vi "obtain_scanner_values.vi"(8 "error in (no error)":errorcluster, 11 "ScanHeadDL090202 in":refnum<class "ScanHeadDL090202.lvclass">) -> (0 "error out":errorcluster, 1 "coerced?":bool[](array[boolean]), 2 "scan signals out":dbl[][](array[numeric]), 3 "ScanHeadDL090202 out":refnum<class "ScanHeadDL090202.lvclass">, 4 "total number of pixels per cycle":i32, 6 "block size":i32)   [LabVIEW 2010, in "ScanHeadDL090202.lvclass"]
uses:
  ScanHeadDL090202.lvclass
  Trajectory/GenericTrajectory/GenericTrajectory/GenericTrajectory.lvclass
  Trajectory/TrajectoryDL091126GenericVoxel/TrajectoryDL091126GenericVoxel/TrajectoryDL091126GenericVoxel.lvclass
  ScanHeadDL090202.lvclass/ScanHeadDL090202.ctl
  Objective/GenericObjective/GenericObjective/GenericObjective.lvclass
  common/classes/ErrorController/ErrorController/class_data.vi
  common/classes/ErrorController/ErrorController/ErrorController.lvclass
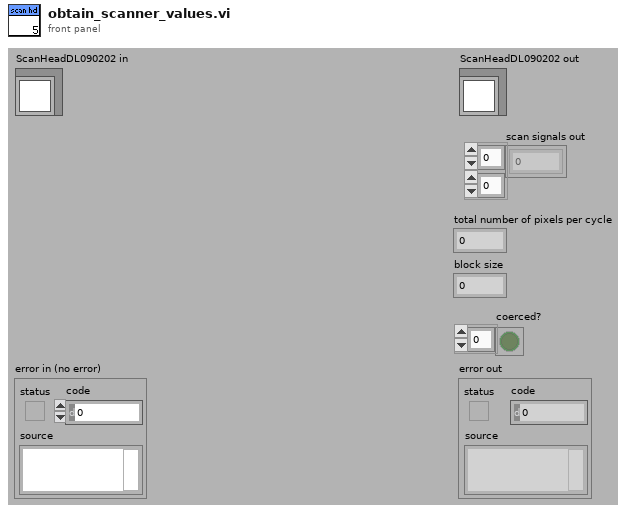
[diagram p1: front panel]
types:
  T1 = typedef "TrajectoryDL091126GenericVoxel.lvclass/transformation_parameters.ctl" = cluster{"scale factor":dbl, "rotation angle":dbl[unit], "tilting angle":dbl[unit], "offset":refnum<class "SpaceVector.lvclass">}
  T2 = cluster{"scanner factors[0]":dbl[unit], "scanner factors[1]":dbl[unit], "scanner factors[2]":dbl[unit]}
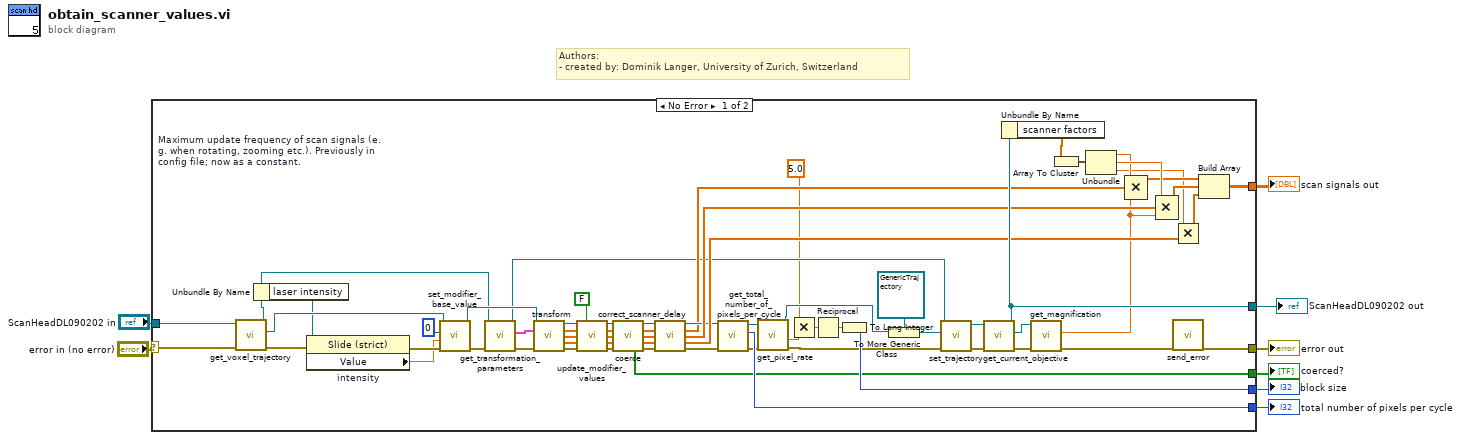
[diagram p0: block diagram]
diagram:
  # "Authors: \n- created by: Dominik Langer, University of Zurich, Switzerland"
  n1 = case shown="No Error" "error in (no error)" {
    selector: "error in (no error)" -> [w18 w75]
    tunnel: [w11 w75] -> w7
    tunnel: [w62 w74] -> w5
    tunnel: "ScanHeadDL090202 in" -> [w71 w74]
    tunnel: [w61 _] -> w4
    tunnel: [w60 _] -> w3
    tunnel: [w47 _] -> w2
    tunnel: [w57 _] -> w1
    frame No Error {
      w9 = dbl[unit] 5.0  # Maximum update frequency of scan signals (e.g. when rotating, zooming etc.). Previously in config file; now as a constant.
      n2 = call-dynamic "get_voxel_trajectory.vi"("error in (no error)"=w18, "ScanHeadDL090202 in"=w71) -> ("error out"=w24:errorcluster, "trajectory"=w52:refnum<class "TrajectoryDL091126GenericVoxel.lvclass">, "ScanHeadDL090202 out"=w20:refnum<class "ScanHeadDL090202.lvclass">)  [unwired: 7 in]
      n3 = Unbundle By Name(w20) -> ("laser intensity"=w48:refnum<vi>)
      n4 = property on="intensity" class="Slide (strict)"(reference=w48, error in=w24) -> (error out=w49:errorcluster, "Value"=w46:dbl)  [unwired: 1 out]
      n5 = call-dynamic "set_modifier_base_value.vi"("error in (no error)"=w49, "modifier base value"=w46, "modifier index"=0, "GenericTrajectory.lvclass in"=w52) -> ("error out"=w23:errorcluster, "GenericTrajectory.lvclass out"=w51:refnum<class "TrajectoryDL091126GenericVoxel.lvclass">)  [unwired: 6 in]
      n6 = call-dynamic "get_transformation_parameters.vi"("error in (no error)"=w23, "ScanHeadDL090202 in"=w20) -> ("error out"=w22:errorcluster, "transformation parameters"=w21:T1, "ScanHeadDL090202 out"=w19:refnum<class "ScanHeadDL090202.lvclass">)  [unwired: 7 in]
      n7 = call-dynamic "transform.vi"("GenericTrajectory in"=w51, "transformation parameters"=w21, "error in (no error)"=w22) -> ("GenericTrajectory out"=w40:refnum<class "TrajectoryDL091126GenericVoxel.lvclass">, "x coordinates"=w42:dbl[unit][], "y coordinates"=w43:dbl[unit][], "z coordinates"=w44:dbl[unit][], "error out"=w45:errorcluster)  [unwired: 8 in]
      n8 = call-dynamic "update_modifier_values.vi"("TrajectoryDL091126GenericVoxel in"=w40, "position-dependently?"=FALSE, "x coordinates in"=w42, "y coordinates in"=w43, "z coordinates in"=w44, "error in (no error)"=w45) -> ("TrajectoryDL091126GenericVoxel out"=w38:refnum<class "TrajectoryDL091126GenericVoxel.lvclass">, "x coordinates out"=w37:dbl[unit][], "y coordindates out"=w36:dbl[unit][], "z coordinates out"=w35:dbl[unit][], "error out"=w39:errorcluster)  [unwired: 5 in]
      n9 = call "coerce.vi"("GenericTrajectory in"=w38, "x coordinates in"=w37, "y coordinates in"=w36, "z coordinates in"=w35, "error in (no error)"=w39) -> ("GenericTrajectory out"=w32:refnum<class "TrajectoryDL091126GenericVoxel.lvclass">, "x coordinates out"=w31:dbl[unit][], "y coordinates out"=w30:dbl[unit][], "z coordinates out"=w29:dbl[unit][], "coerced?"=w47:bool[], "error out"=w34:errorcluster)  [unwired: 5 in]
      n10 = call-dynamic "correct_scanner_delay.vi"("TrajectoryDL091126GenericVoxel in"=w32, "x coordinates in"=w31, "y coordinates in"=w30, "z coordinates in"=w29, "error in (no error)"=w34) -> ("TrajectoryDL091126GenericVoxel out"=w26:refnum<class "TrajectoryDL091126GenericVoxel.lvclass">, "x coordinates out"=w25:dbl[unit][], "y coordinates out"=w27:dbl[unit][], "z coordinates out"=w28:dbl[unit][], "error out"=w33:errorcluster)  [unwired: 6 in]
      n11 = call-dynamic "get_total_number_of_pixels_per_cycle.vi"("error in (no error)"=w33, "GenericTrajectory in"=w26) -> ("error out"=w17:errorcluster, "total number of pixels per cycle"=w61:i32, "GenericTrajectory out"=w16:refnum<class "TrajectoryDL091126GenericVoxel.lvclass">)  [unwired: 7 out]
      n12 = call-dynamic "get_pixel_rate.vi"("error in (no error)"=w17, "GenericTrajectory in"=w16) -> ("error out"=w14:errorcluster, "pixel dwell time"=w13:dbl[unit], "GenericTrajectory out"=w15:refnum<class "TrajectoryDL091126GenericVoxel.lvclass">)  [unwired: 6 in, 1 out]
      n13 = Multiply(x=w9, y=w13) -> (x*y=w73:dbl)
      n14 = Reciprocal(x=w73) -> (1/x=w72:dbl)
      n15 = To Long Integer(number=w72) -> (32bit integer=w60:i32)
      n16 = To More Generic Class(target class=refnum<class "GenericTrajectory.lvclass"> refnum ("GenericTrajectory.lvclass"), reference=w15) -> (generic class reference=w53:refnum<class "GenericTrajectory.lvclass">)
      n17 = call-dynamic "set_trajectory.vi"("error in (no error)"=w14, "trajectory"=w53, "GenericScanHead.lvclass in"=w19) -> ("error out"=w56:errorcluster, "GenericScanHead.lvclass out"=w55:refnum<class "ScanHeadDL090202.lvclass">)  [unwired: 7 in]
      n18 = call-dynamic "get_current_objective.vi"("error in (no error)"=w56, "GenericPlugin in"=w55) -> ("error out"=w69:errorcluster, "current objective"=w70:refnum<class "GenericObjective.lvclass">, "GenericPlugin out"=w62:refnum<class "ScanHeadDL090202.lvclass">)  [unwired: 7 in]
      n19 = Unbundle By Name(w62) -> ("scanner factors"=w65:dbl[unit][])
      n20 = call-dynamic "get_magnification.vi"("error in (no error)"=w69, "GenericObjective in"=w70) -> ("error out"=w12:errorcluster, "magnification"=w10:dbl)  [unwired: 7 in, 1 out]
      n21 = Array To Cluster(array=w65) -> (cluster=w64:T2)
      n22 = Unbundle(w64) -> ("scanner factors[0]"=w66:dbl[unit], "scanner factors[1]"=w67:dbl[unit], "scanner factors[2]"=w59:dbl[unit])
      n23 = Compound Arithmetic op=MULTIPLY(w66, w25, w10) -> (w63:dbl[])
      n24 = Compound Arithmetic op=MULTIPLY(w67, w27, w10) -> (w68:dbl[])
      n25 = Multiply(x=w59, y=w28) -> (x*y=w58:dbl[])
      n26 = call "send_error.vi"("error in (no error)"=w12) -> ("error out"=w11:errorcluster)  [unwired: 10 in]
      n27 = Build Array(w63, w68, w58) -> (w57:dbl[][])
    }
    frame Error {
    }
  }
  "error out" <- w7
  "ScanHeadDL090202 out" <- w5
  "scan signals out" <- w1
  "total number of pixels per cycle" <- w4
  "block size" <- w3
  "coerced?" <- w2
